vi "configuration_microphone.vi"() -> (3 "configuration_microphone":T1={"chunk"=512, "profile"=3, "level"=41, "_reserved_0"=0, "_reserved_1"=0, "_reserved_2"=0, "_reserved_3"=0, "_reserved_4"=0, "_reserved_5"=0})   [LabVIEW 2023]
panel:
  in  "configuration_microphone":T1={"chunk"=512, "profile"=3, "level"=41, "_reserved_0"=0, "_reserved_1"=0, "_reserved_2"=0, "_reserved_3"=0, "_reserved_4"=0, "_reserved_5"=0}
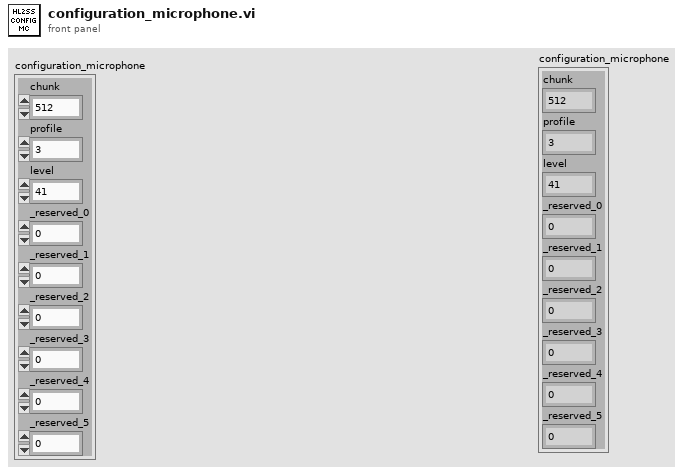
[diagram p1: front panel]
types:
  T1 = cluster{"chunk":u64, "profile":u8, "level":u8, "_reserved_0":u8, "_reserved_1":u8, "_reserved_2":u8, "_reserved_3":u8, "_reserved_4":u8, "_reserved_5":u8}
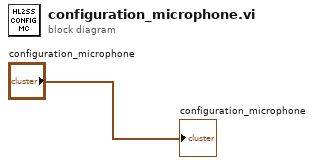
[diagram p0: block diagram]
diagram:
  "configuration_microphone" <- "configuration_microphone"
